vi "StopwatchSub.vi"(10 "Reset":bool) -> (2 "Time(Seconds)":dbl)   [LabVIEW 2018]
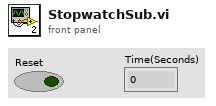
[diagram p1: front panel]
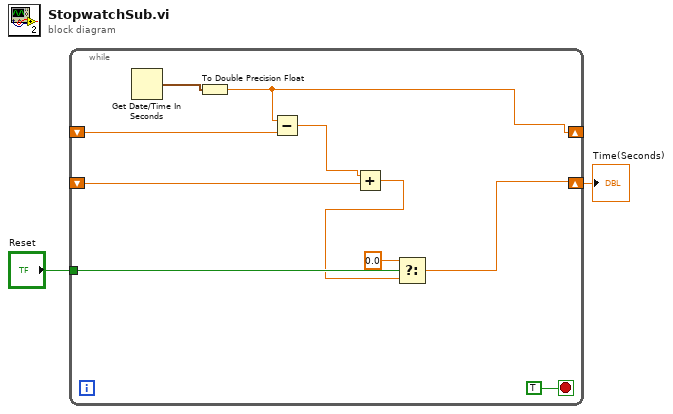
[diagram p0: block diagram]
diagram:
  n1 = while {
    shift-right: [w10] -> _
    shift-left: _ -> [w11]
    shift-right: [w4] -> w2
    shift-left: _ -> [w9]
    tunnel: "Reset" -> [w7]
    stop <- TRUE stop-if-true
    n2 = Get Date/Time In Seconds() -> (seconds since 1Jan1904=w12:timestamp)
    n3 = To Double Precision Float(number=w12) -> (double precision float=w10:dbl)
    n4 = Subtract(x=w10, y=w11) -> (x-y=w8:dbl)
    n5 = Add(x=w8, y=w9) -> (x+y=w5:dbl)
    n6 = Select(t=0.0, s=w7, f=w5) -> (s? t:f=w4:dbl)
  }
  "Time(Seconds)" <- w2
